vi "Wait for Host.vi"(8 "error in":errorcluster, 9 "STM queue":refnum<queue>, 11 "local tcp port":u16=61558) -> (0 "error out":errorcluster, 3 "connection ID":refnum<k5>)   [LabVIEW 2017, in "WinHost.lvlib"]
uses:
  WinHost.lvlib
  Private TypeDefs/STM Queue Element.ctl
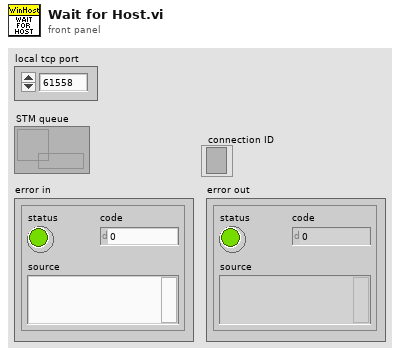
[diagram p1: front panel]
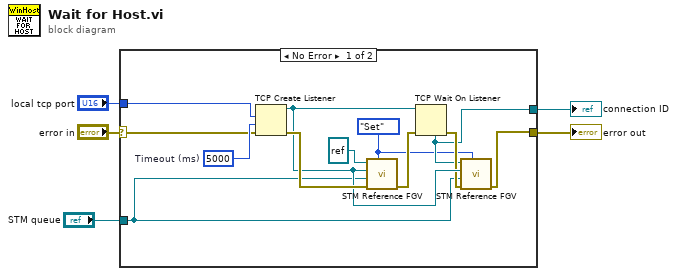
[diagram p0: block diagram]
diagram:
  n1 = case shown="No Error" "error in" {
    selector: "error in" -> [w10 w18]
    tunnel: "local tcp port" -> [w15 _]
    tunnel: [w9 w18] -> w3
    tunnel: [w8 _] -> w2
    tunnel: "STM queue" -> [w6 _]
    frame No Error {
      w7 = enum16{"Set", "Get"}."Set" ("Command")
      w14 = 5000  # Timeout (ms)
      n2 = TCP Create Listener(8:w10, 9:w14, 10:w15) -> (0:w17:errorcluster, 3:w13:refnum<k5>)  [unwired: 2 in, 1 out]
      n3 = call "STM Reference FGV.vi"("command"=w7, "error in"=w17, "STM queue in"=w6, "TCP listener ID in"=w13, "TCP connection ID in"=refnum<k5> refnum ("TCP Connection ID")) -> ("error ou"=w12:errorcluster)  [unwired: 3 in, 3 out]
      n4 = TCP Wait On Listener(8:w12, 11:w13) -> (0:w11:errorcluster, 4:w8:refnum<k5>)  [unwired: 2 in, 3 out]
      n5 = call "STM Reference FGV.vi"("command"=w7, "error in"=w11, "STM queue in"=w6, "TCP listener ID in"=w13, "TCP connection ID in"=w8) -> ("error ou"=w9:errorcluster)  [unwired: 3 in, 3 out]
    }
    frame Error {
    }
  }
  "error out" <- w3
  "connection ID" <- w2
